vi "MSOConfig.vi"(0 "object in":refnum<class "AD2_MSO_SDK.lvclass">, 2 "Config":T1={"Timing"={"Enable"=TRUE, "Samples In"=0.0, "Sample Rate"=0.0, "Mode"=enum."Single Sample"}, "Trigger"={"Hysteresis"=0.0, "Trigger Level"=0.0, "Trigger Condition"=0, "Trigger Type"=0, "Trigger Channel"=0, "secTimeout"=0.0, "TrigrSrc"=enum."trigrsrcNone"}, "Range Ch1"={"idxChannel"=0, "voltOffset"=0.0, "VoltsRange"=0}, "Range Ch 2"={"idxChannel"=0, "voltOffset"=0.0, "VoltsRange"=0}} {"Range Ch 2"."VoltsRange" items=["High 50V"=50, "Low5V"=5]; "Range Ch1"."VoltsRange" items=["High 50V"=50, "Low5V"=5]; "Trigger"."Trigger Channel" items=["Channel 1"=0, "Channel 2"=1, "Both"=-1]; "Trigger"."Trigger Type" items=["Edge", "Pulse", "Transition"]; "Trigger"."Trigger Condition" items=["Rising", "Falling"]}, 5 "error in (no error)":errorcluster) -> (14 "object out":refnum<class "AD2_MSO_SDK.lvclass">, 19 "error out":errorcluster)   [LabVIEW 2023, in "AD2_MSO_SDK.lvclass"]
uses:
  AD2_MSO_SDK.lvclass
  MSOConfig.ctl
  AD2TriggerSources.ctl
  MSORangeCh.ctl
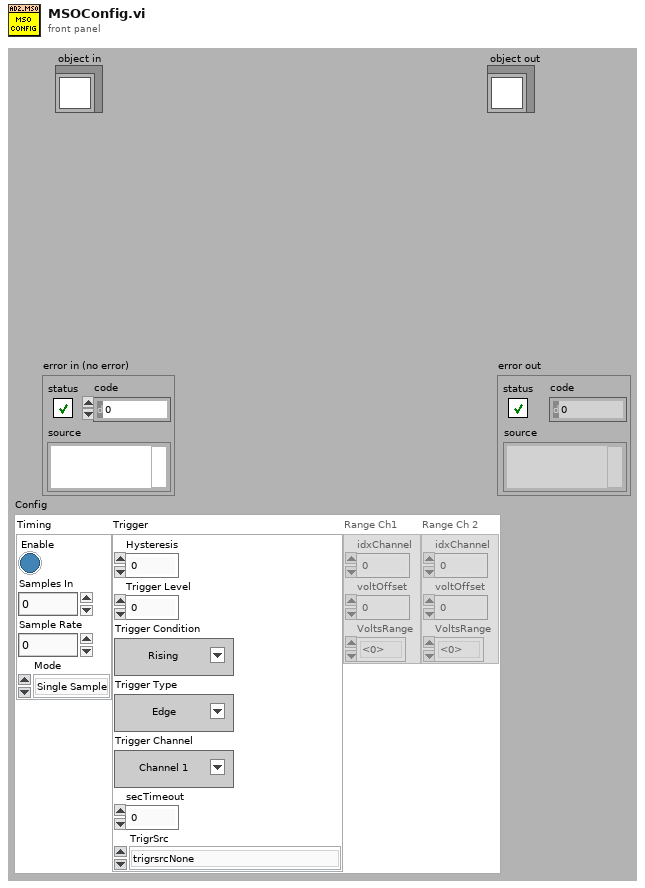
[diagram p1: front panel]
types:
  T1 = typedef "AD2_MSO_SDK.lvclass/MSOConfig.ctl" = cluster{"Timing":cluster{"Enable":bool, "Samples In":dbl, "Sample Rate":dbl, "Mode":enum16{"Single Sample", "Scanshift", "Multiple Samples", "Scan Screen"}}, "Trigger":cluster{"Hysteresis":dbl, "Trigger Level":dbl, "Trigger Condition":i32, "Trigger Type":i32, "Trigger Channel":i32, "secTimeout":dbl, "TrigrSrc":T2}, "Range Ch1":T3, "Range Ch 2":T3}
  T2 = typedef "AD2_MSO_SDK.lvclass/AD2TriggerSources.ctl" = enum8{"trigrsrcNone", "trigsrcPC", "trigsrcDetectorAnalogIn", "trigsrcDetectorDigitalIn", "trigsrcAnalogIn", "trigsrcDigitalIn", "trigsrcDigitalOut", "trigsrcAnalogOut1", "trigsrcAnalogOut2", "trigsrcAnalogOut3", "trigsrcAnalogOut4", "trigsrcExternal1", "trigsrcExternal2", "trigsrcExternal3", "trigsrcExternal4", ""}
  T3 = typedef "AD2_MSO_SDK.lvclass/MSORangeCh.ctl" = cluster{"idxChannel":i32, "voltOffset":dbl, "VoltsRange":u16}
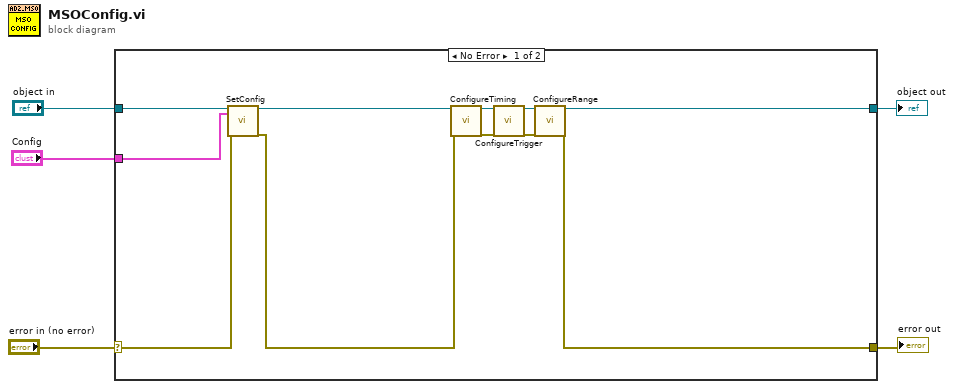
[diagram p0: block diagram]
diagram:
  n1 = case shown="No Error" "error in (no error)" {
    selector: "error in (no error)" -> [w7 w18]
    tunnel: [w11 w18] -> w4
    tunnel: [w14 w17] -> w2
    tunnel: "object in" -> [w9 w17]
    tunnel: "Config" -> [w8 _]
    frame No Error {
      n2 = call-dynamic "SetConfig.vi"("object in"=w9, "Config"=w8, "error in (no error)"=w7) -> ("object out"=w10:refnum<class "AD2_MSO_SDK.lvclass">, "error out"=w6:errorcluster)  [unwired: 15 in]
      n3 = call-dynamic "ConfigureTiming.vi"("object in"=w10, "error in (no error)"=w6) -> ("object out"=w16:refnum<class "AD2_MSO_SDK.lvclass">, "error out"=w13:errorcluster)  [unwired: 16 in]
      n4 = call-dynamic "ConfigureTrigger.vi"("object in"=w16, "error in (no error)"=w13) -> ("object out"=w15:refnum<class "AD2_MSO_SDK.lvclass">, "error out"=w12:errorcluster)  [unwired: 16 in]
      n5 = call-dynamic "ConfigureRange.vi"("object in"=w15, "error in (no error)"=w12) -> ("object out"=w14:refnum<class "AD2_MSO_SDK.lvclass">, "error out"=w11:errorcluster)  [unwired: 16 in]
    }
    frame Error {
    }
  }
  "error out" <- w4
  "object out" <- w2
